vi "Check for Wheel Type Match.vi"(5 "chain levels to remove (2)":i32=2, 7 "produce warning if no match (T)":bool=TRUE, 8 "error in (no error)":errorcluster, 10 "target wheel type":refnum<class "NI_Robotics_Wheel.lvclass">, 11 "wheel in":refnum<class "NI_Robotics_Wheel.lvclass">) -> (0 "error out":errorcluster, 2 "match?":bool, 3 "wheel out":refnum<class "NI_Robotics_Wheel.lvclass">)   [LabVIEW 2017, in "NI_Robotics_Wheel.lvclass"]
uses:
  <vilib>/robotics/Steering/Wheel/NI_Robotics_Wheel.lvclass
  <vilib>/robotics/Utilities/NI_Robotics Utilities.lvlib
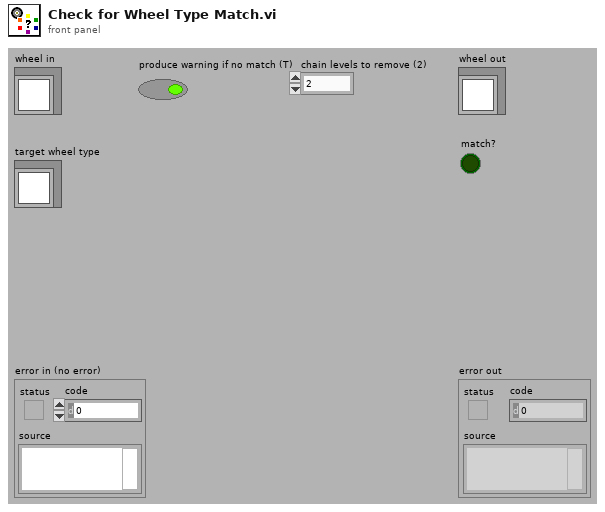
[diagram p1: front panel]
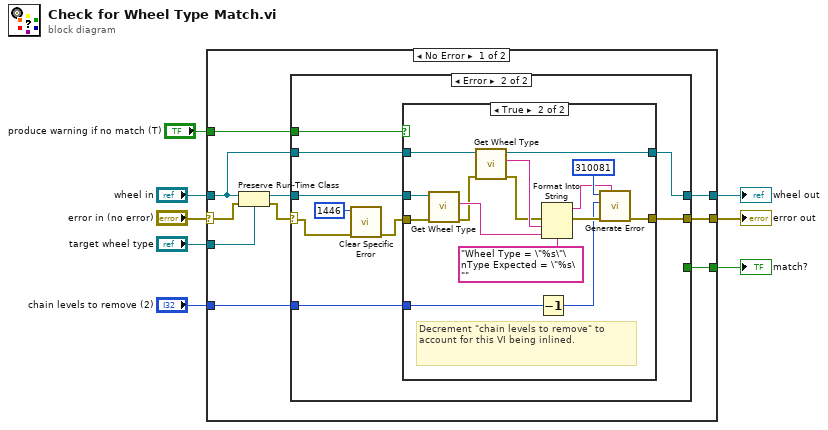
[diagram p0: block diagram]
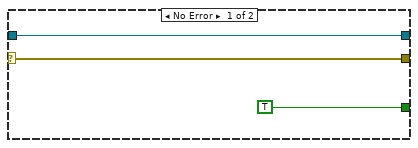
[diagram p2: hidden frame]
diagram:
  n1 = case shown="No Error" "error in (no error)" {
    selector: "error in (no error)" -> [w18 w49]
    tunnel: [w14 w49] -> w7
    tunnel: [w15 w48] -> w5
    tunnel: "wheel in" -> [w11 w48]
    tunnel: "target wheel type" -> [w9 _]
    tunnel: "produce warning if no match (T)" -> [w12 _]
    tunnel: [w13 _] -> w2
    tunnel: "chain levels to remove (2)" -> [w10 _]
    frame No Error {
      n2 = Preserve Run-Time Class(object in=w11, error in=w18, 2:w9) -> (object out=w16:refnum<class "NI_Robotics_Wheel.lvclass">, error out=w17:errorcluster)
      n3 = case shown="Error" w17 {
        selector: w17 -> [w20 w24]
        tunnel: w16 -> [w21 w27]
        tunnel: [w21 w29] -> w15
        tunnel: [w20 w28] -> w14
        tunnel: w11 -> [_ w30]
        tunnel: [TRUE _] -> w13
        tunnel: w12 -> [_ w26]
        tunnel: w10 -> [_ w25]
        frame No Error {
        }
        frame Error {
          n4 = call <vilib>:"Clear Specific Error.vi"("error in (no error)"=w24, "code"=1446) -> ("error out"=w23:errorcluster)  [unwired: 7 in, 2 out]
          n5 = case shown="True" w26 {
            tunnel: w30 -> [w32 w42]
            tunnel: [w32 w41] -> w29
            tunnel: [w31 w40] -> w28
            tunnel: w27 -> [_ w38]
            tunnel: w25 -> [_ w35]
            tunnel: w23 -> [w31 w34]
            frame False {
            }
            frame True {
              # "Decrement \"chain levels to remove\" to account for this VI being inlined."
              n6 = call-dynamic "Get Wheel Type.vi"("error in (no error)"=w34, "wheel in"=w38) -> ("error out"=w43:errorcluster, "wheel type"=w47:string)  [unwired: 7 in, 1 out]
              n7 = call-dynamic "Get Wheel Type.vi"("error in (no error)"=w43, "wheel in"=w42) -> ("error out"=w44:errorcluster, "wheel type"=w46:string, "wheel out"=w41:refnum<class "NI_Robotics_Wheel.lvclass">)  [unwired: 7 in]
              n8 = Decrement(x=w35) -> (x-1=w33:i32)
              n9 = Format Into String(format string="Wheel Type = \"%s\"\nType Expected = \"%s\"", error in=w44, w46, w47) -> (resulting string=w37:string, error out=w36:errorcluster)  [unwired: 1 in]
              n10 = call <vilib>:"Generate Error.vi"("<append> (\"\")"=w37, "error in (no error)"=w36, "chain levels to remove (1)"=w33, "code"=310081) -> ("error out"=w40:errorcluster)  [unwired: 7 in]
            }
          }
        }
      }
    }
    frame Error {
    }
  }
  "error out" <- w7
  "wheel out" <- w5
  "match?" <- w2
